vi "Experiments UI.vi"() -> ()   [LabVIEW 2009, in "UI.lvlib"]
uses:
  UI.lvlib
  database/Experiment.ctl
  database/Block.ctl
  Close Notification.vi
  database/Data Store.lvclass
  database/Database.lvlib
  time/Time.lvlib
panel:
  out "Current Block":T1
  in  "Edit users":bool
  out "Experiment status":string
  in  "Save changes":bool
  out "error out":errorcluster
  in  "Run expt":bool
  in  "Description":string
  in  "Name":string
  in  "Update listbox":bool
  out "Working Set":T2[](array[typedef])
  in  "Reload Working Set":bool
  in  "Update Editor":bool
  in  "Delete":bool
  out "Date/time created":string
  in  "New Experiment":bool
  in  "User":u16(ring)=1 items=["CCLDAS"=1, "LDEX"=2]
  in  "Experiments":i32(listbox)
  # "\"Running\" means all dust events will be marked as belonging to this experiment. \nYou can start and stop the experiment as often as you want."
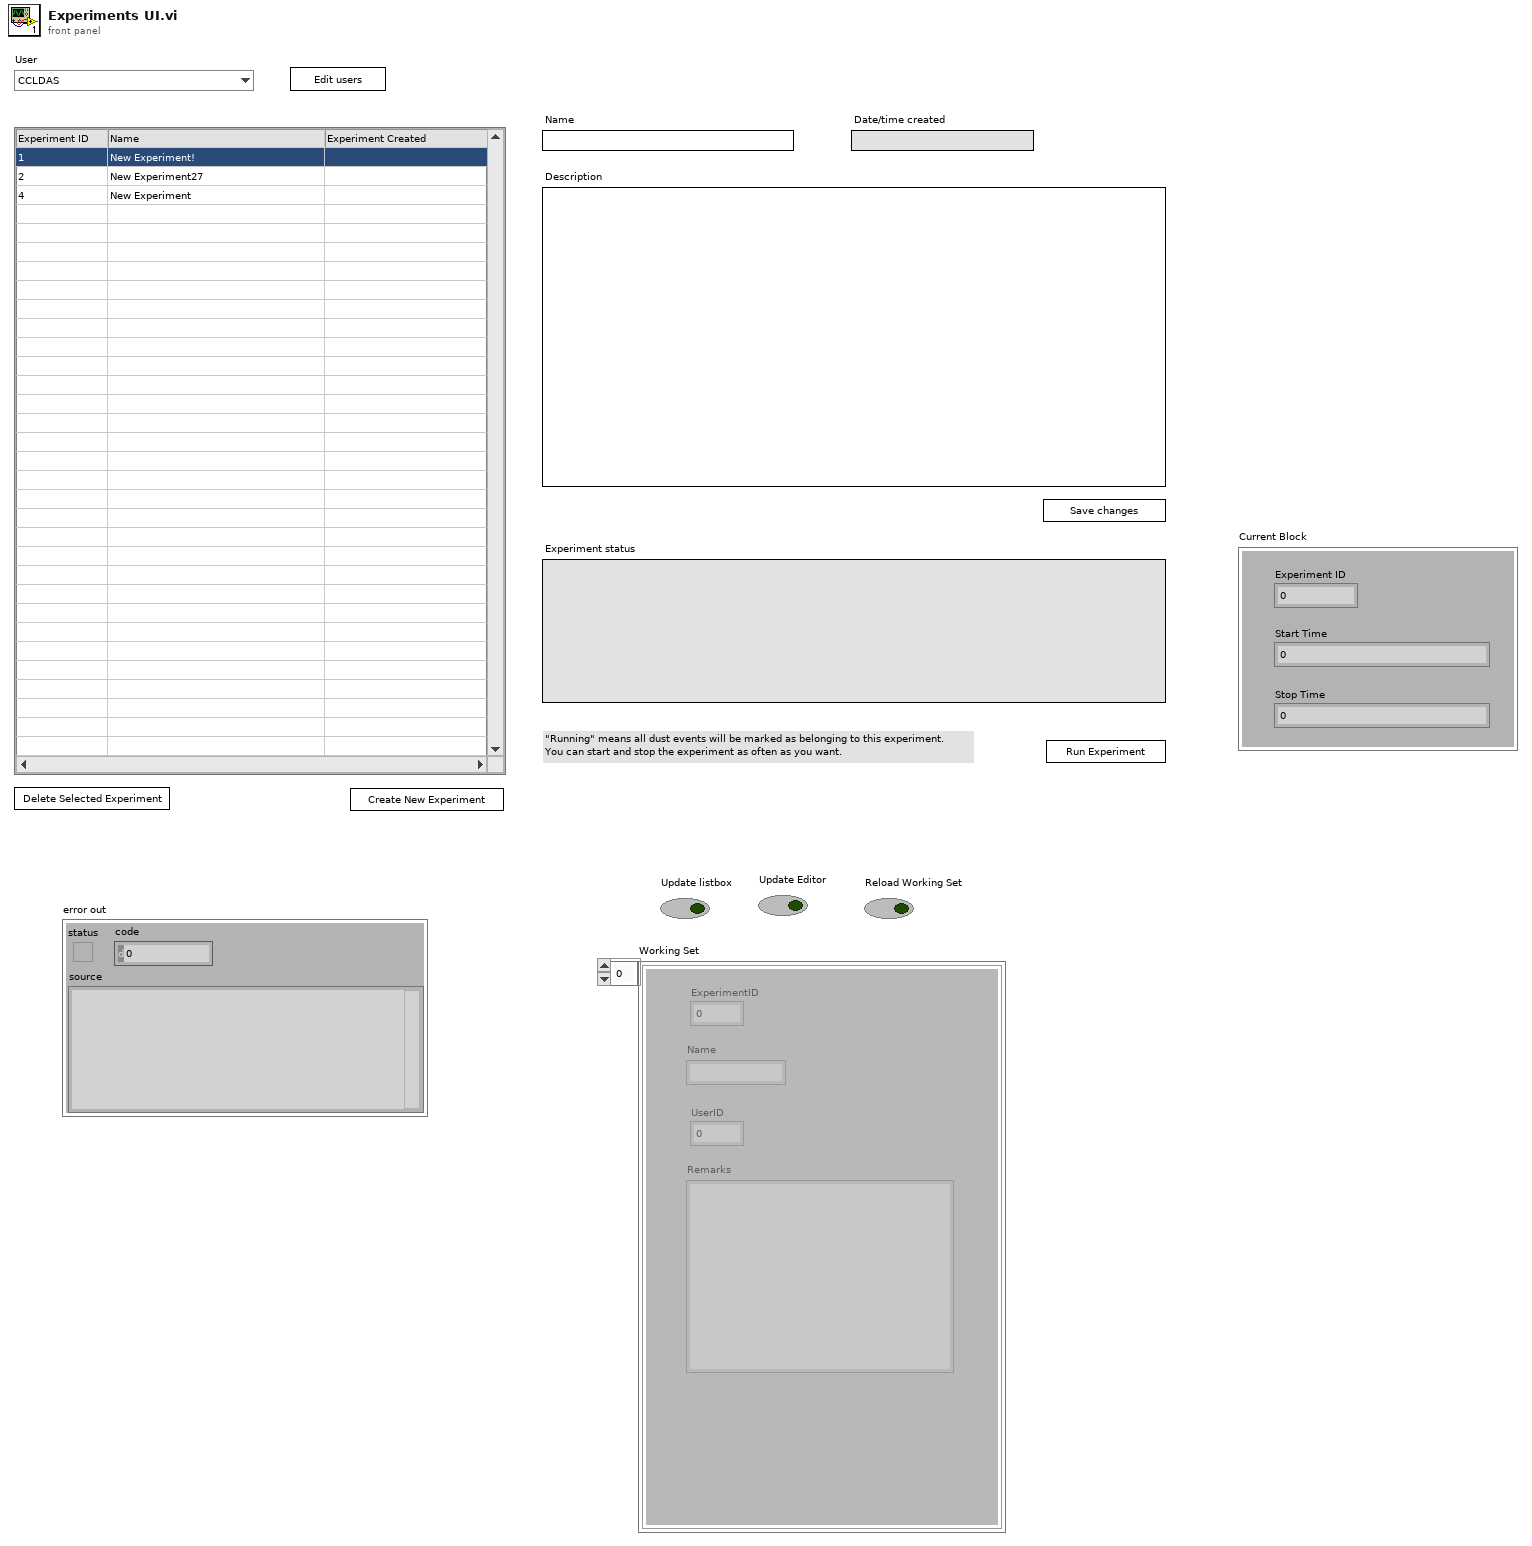
[diagram p1: front panel]
types:
  T1 = typedef "Database.lvlib/Block.ctl" = cluster{"Experiment ID":i32, "Start Time":u64, "Stop Time":u64}
  T2 = typedef "Database.lvlib/Experiment.ctl" = cluster{"ExperimentID":i32, "Name":string, "UserID":i32, "Remarks":string}
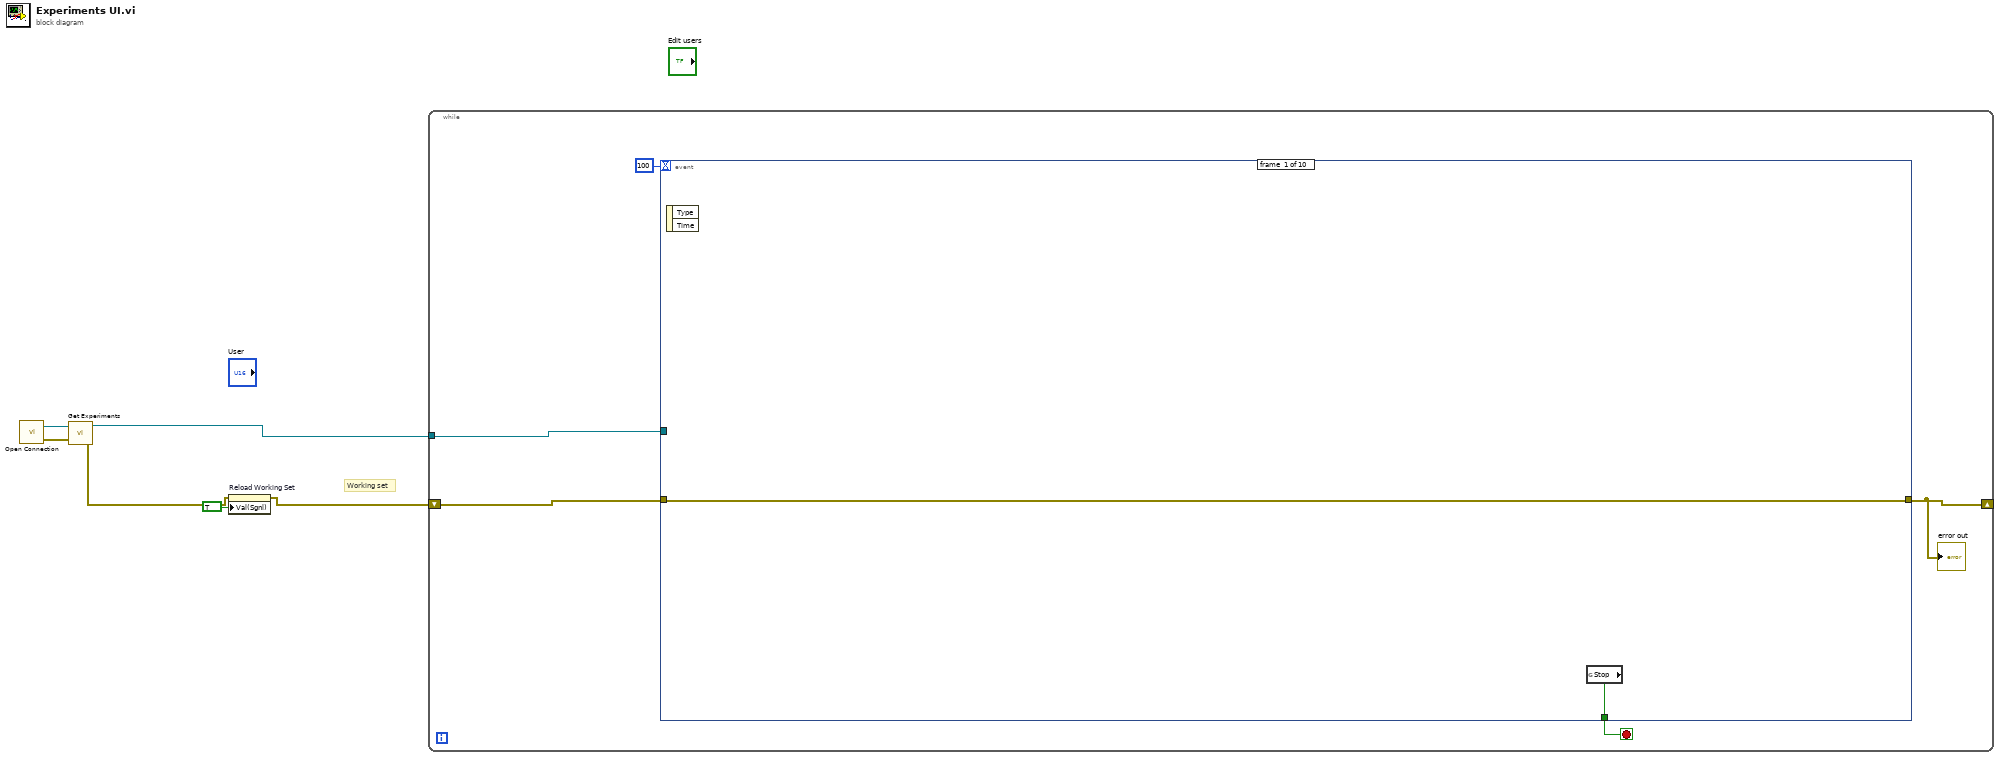
[diagram p0: block diagram]
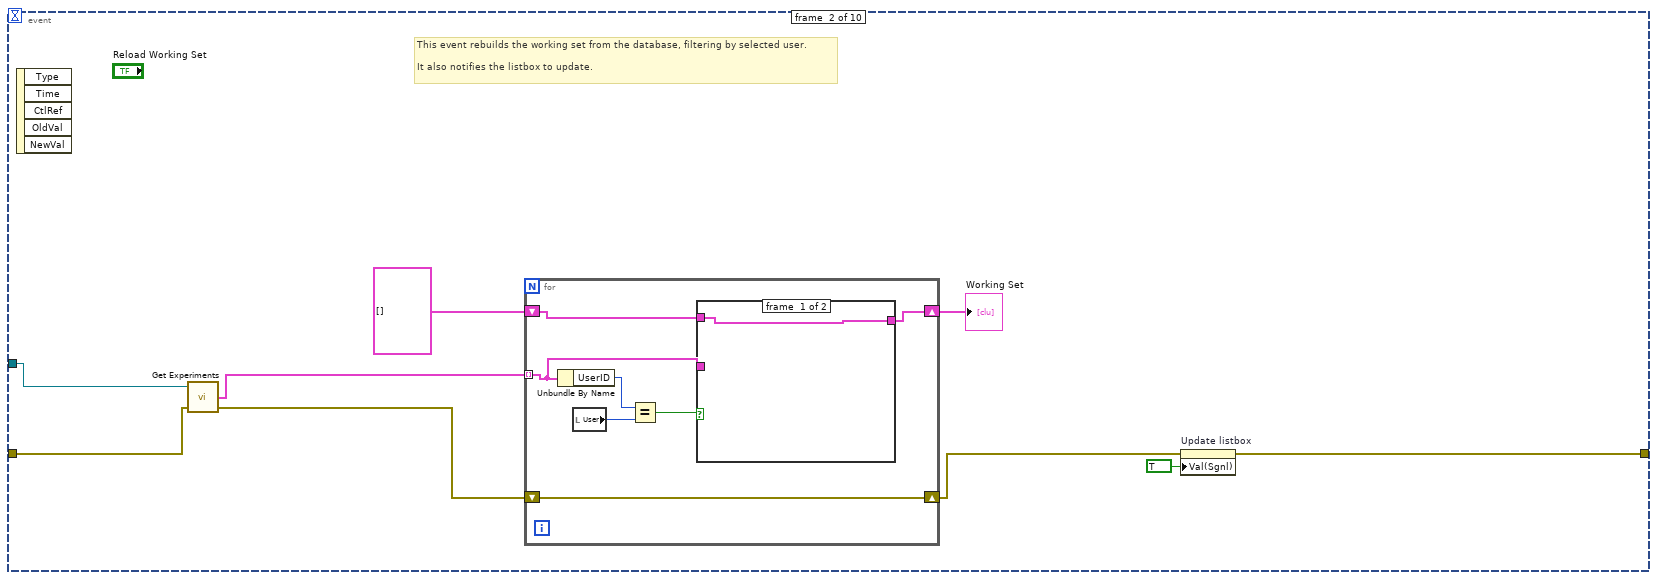
[diagram p2: hidden frame]
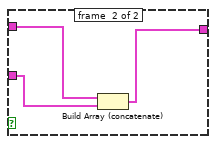
[diagram p3: hidden frame]
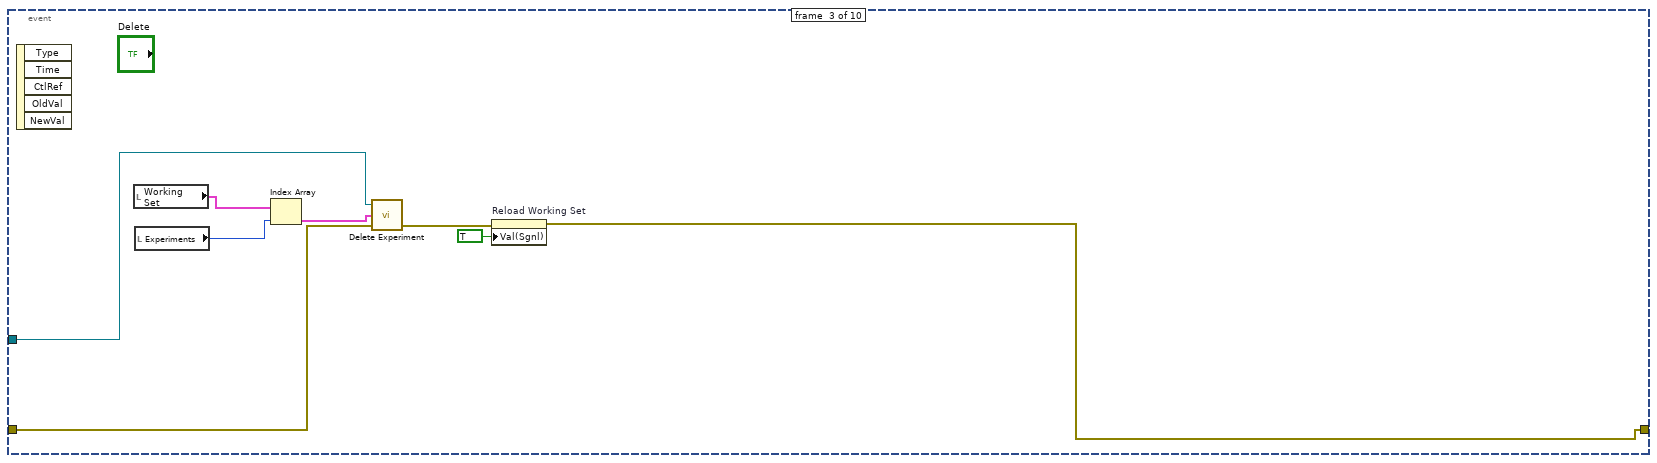
[diagram p4: hidden frame]
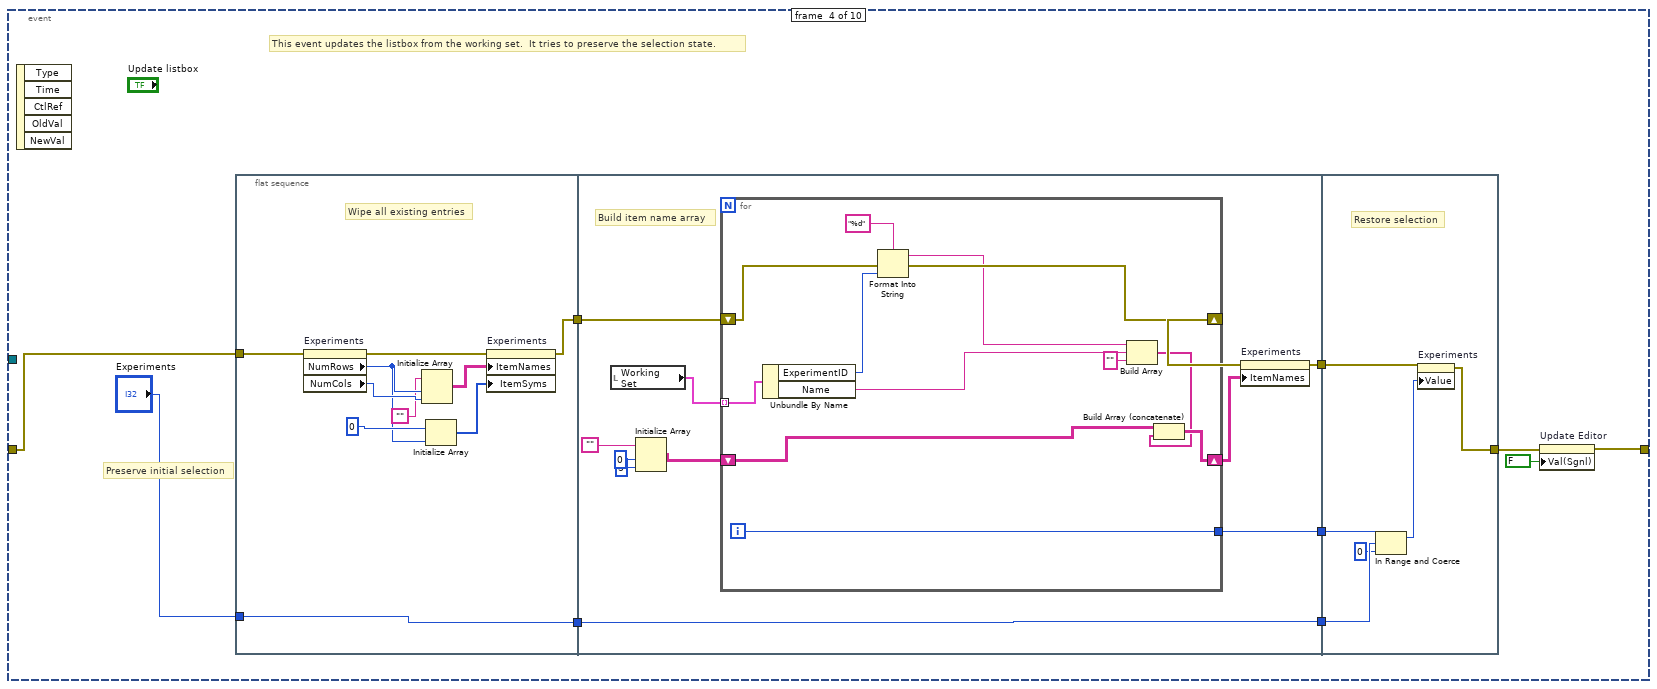
[diagram p5: hidden frame]
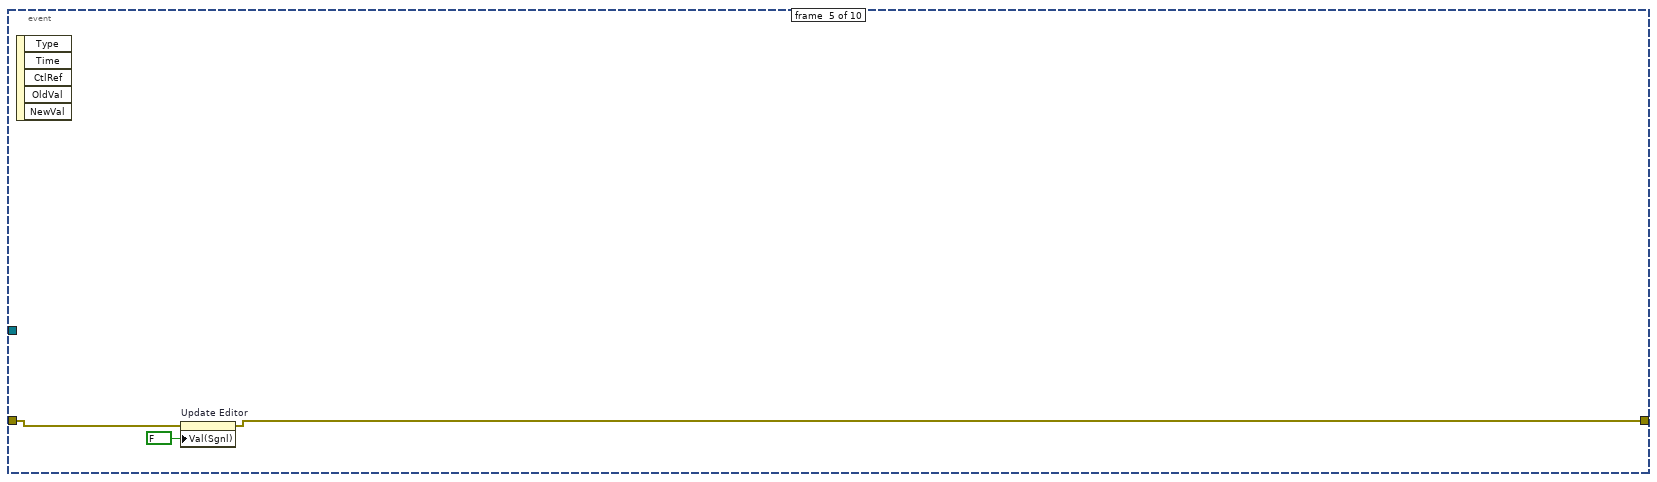
[diagram p6: hidden frame]
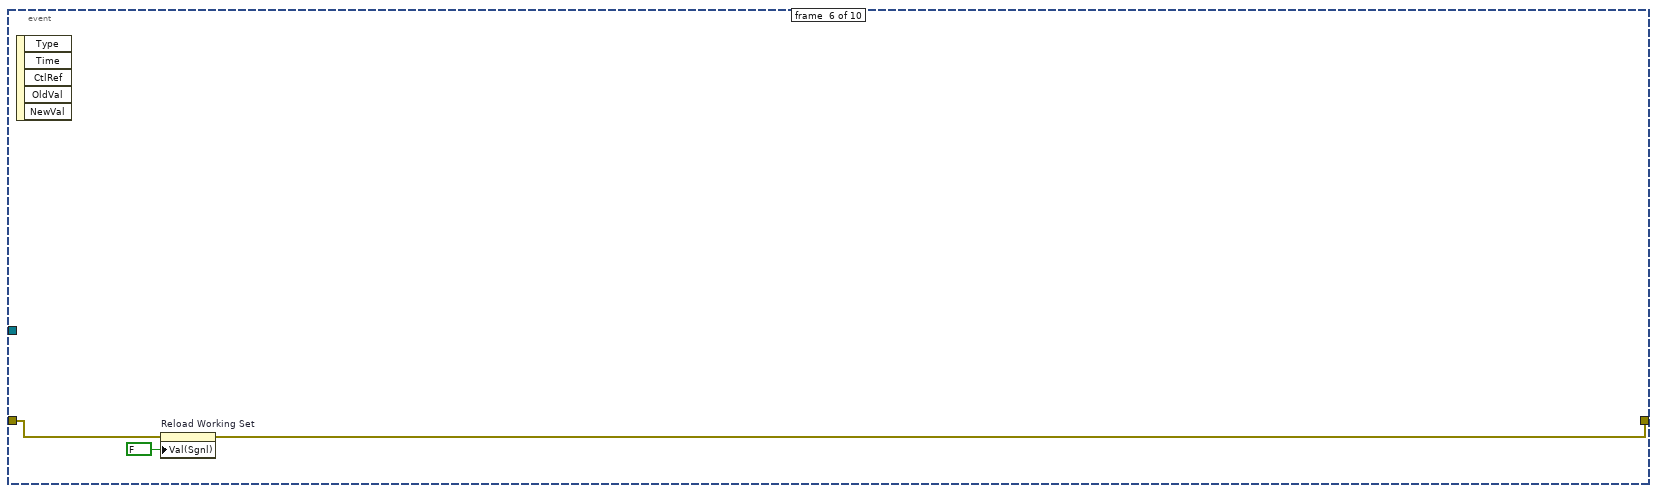
[diagram p7: hidden frame]
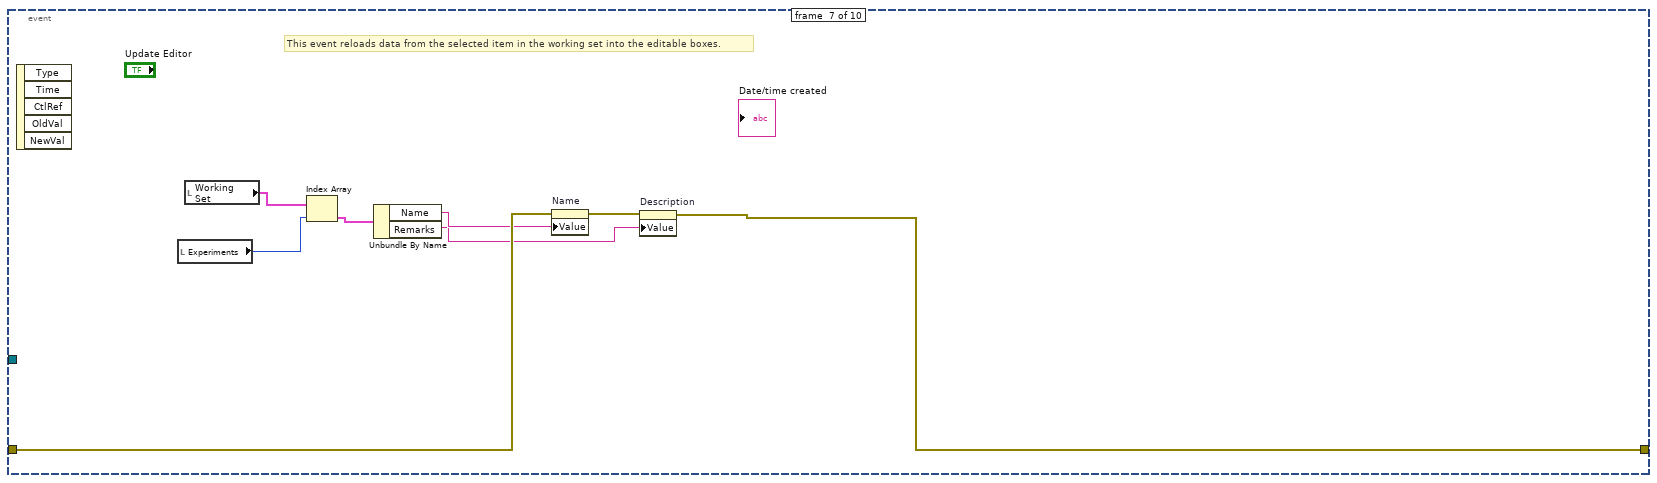
[diagram p8: hidden frame]
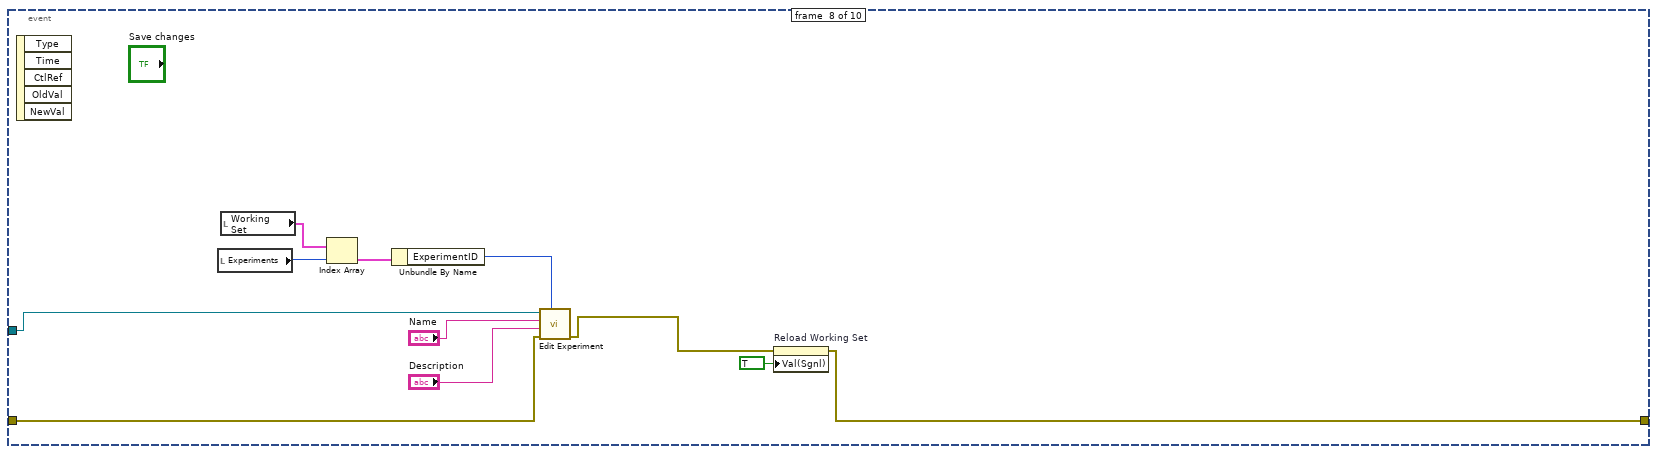
[diagram p9: hidden frame]
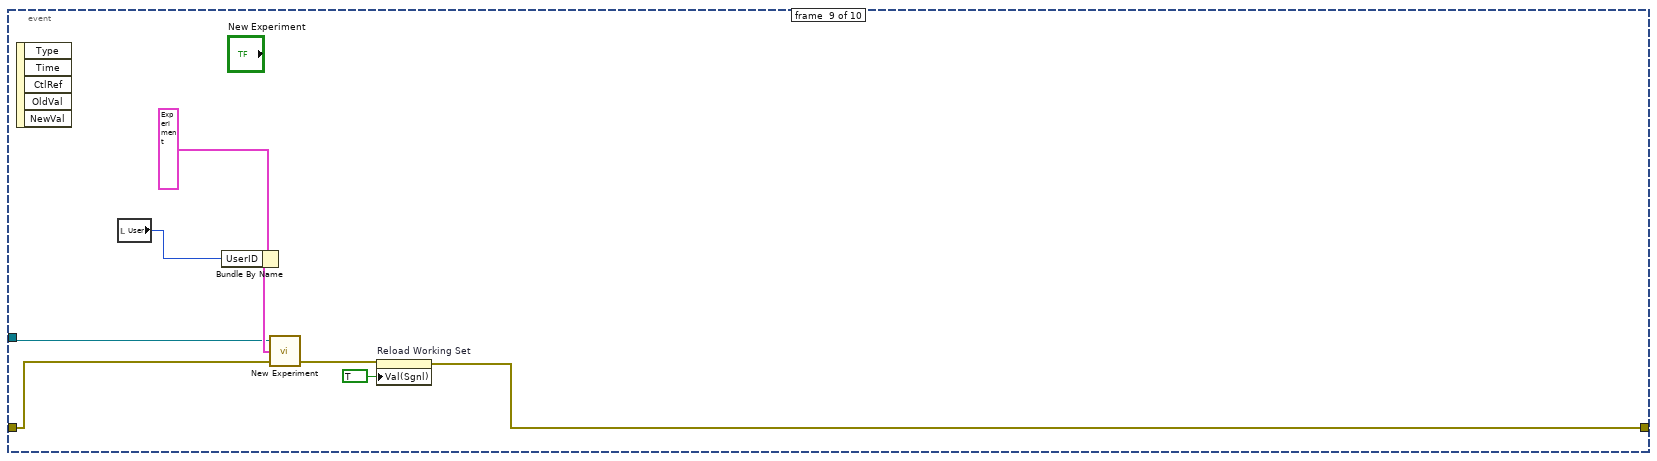
[diagram p10: hidden frame]
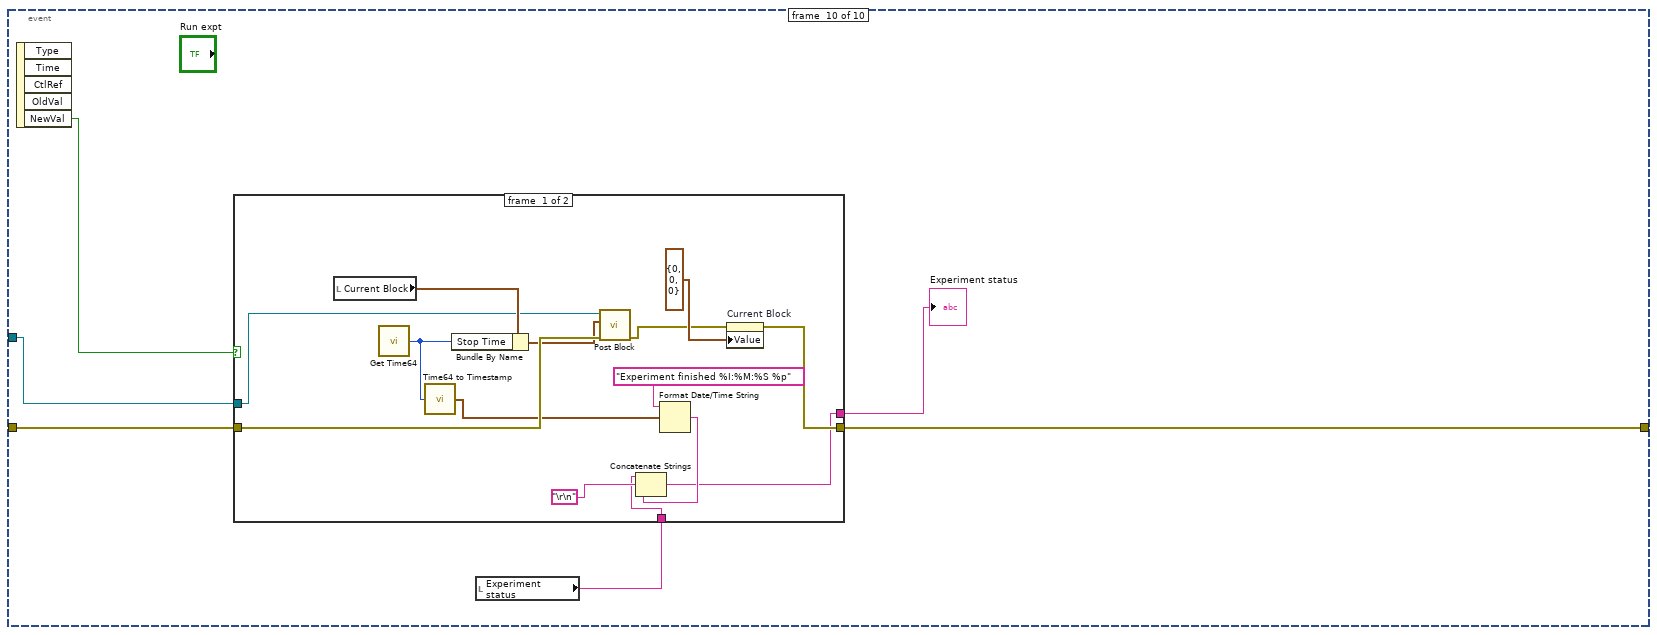
[diagram p11: hidden frame]
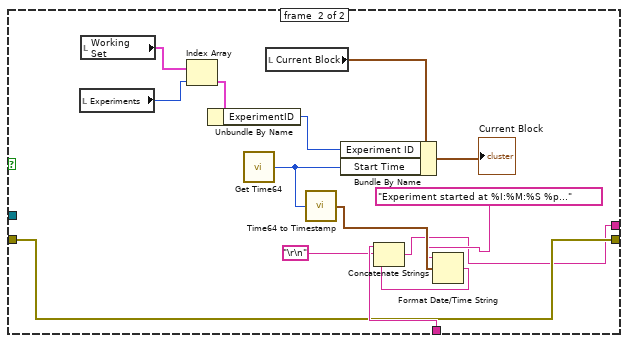
[diagram p12: hidden frame]
diagram:
  # "Working set"
  n1 = call "Open Connection.vi"() -> ("error out"=w6:errorcluster, "Database.lvlib:Data Store.lvclass"=w5:refnum<class "Data Store.lvclass">)  [unwired: 2 in]
  n2 = call "Get Experiments.vi"("error in (no error)"=w6, "Database.lvlib:Data Store.lvclass"=w5) -> ("error out"=w3:errorcluster, "Database.lvlib:Data Store.lvclass 2"=w4:refnum<class "Data Store.lvclass">)  [unwired: 1 in, 1 out]
  n3 = property on="Reload Working Set" class="Bool (strict)"(error in=w3, "Val(Sgnl)"=TRUE ("Value (Signaling)")) -> (error out=w2:errorcluster)  [unwired: 1 in, 1 out]
  n4 = while {
    shift-right: [w7] -> _
    shift-left: w2 -> [w11]
    tunnel: w4 -> [w10]
    stop <- w8 stop-if-true
    n5 = event shown="[9] \"Run expt\": Value Change" {
      selector: _ -> [_ _ _ _ _ _ _ _ _ _]
      dyn-events: _ -> [_ _ _ _ _ _ _ _ _ _]
      timeout: 100 -> [_ _ _ _ _ _ _ _ _ _]
      tunnel: w11 -> [w13 w22 w37 w50 w93 w95 w101 w114 w120 w128]
      tunnel: [w13 w20 w35 w43 w91 w94 w97 w107 w116 w127] -> w7
      tunnel: w10 -> [_ w21 w39 _ _ _ _ w115 w119 w126]
      tunnel: [w12 _ _ _ _ _ _ _ _ _] -> w8
      event #0 {
        n6 = event-data() -> ()  [unwired: 1 in, 2 out]
        n7 = global read "Close Notification.vi" "Stop"() -> (w12:bool)
      }
      event #1 {
        # "This event rebuilds the working set from the database, filtering by selected user.\n\nIt also notifies the listbox to update."
        n8 = event-data() -> ()  [unwired: 1 in, 5 out]
        n9 = call "Get Experiments.vi"("error in (no error)"=w22, "Database.lvlib:Data Store.lvclass"=w21) -> ("error out"=w16:errorcluster, "Array"=w15:T2[])  [unwired: 1 in, 1 out]
        n10 = for {
          shift-right: [w26] -> w17
          shift-left: T2[] [] ("Working Set") -> [w27]
          shift-right: [w23] -> w14
          shift-left: w16 -> [w23]
          tunnel: w15 -> [w24] mode=indexing
          n11 = Unbundle By Name(w24) -> ("UserID"=w29:i32)
          n12 = local read "User"() -> (w28:u16)
          n13 = Equal?(x=w29, y=w28) -> (x = y?=w25:bool)
          n14 = case shown="True" w25 {
            tunnel: w27 -> [w30 w33]
            tunnel: [w30 w31] -> w26
            tunnel: w24 -> [_ w32]
            frame #0 {
            }
            frame #1 {
              n15 = Build Array (concatenate)(w33, w32) -> (w31:T2[])
            }
          }
        }
        "Working Set" <- w17
        n16 = property on="Update listbox" class="Bool (strict)"(error in=w14, "Val(Sgnl)"=TRUE ("Value (Signaling)")) -> (error out=w20:errorcluster)  [unwired: 1 in, 1 out]
      }
      event #2 {
        n17 = event-data() -> ()  [unwired: 1 in, 5 out]
        n18 = local read "Working Set"() -> (w41:T2[])
        n19 = local read "Experiments"() -> (w40:i32)
        n20 = Index Array(array=w41, index=w40) -> (element=w38:T2)
        n21 = call "Delete Experiment.vi"("error in (no error)"=w37, "Experiment to Delete"=w38, "Database.lvlib:Data Store.lvclass"=w39) -> ("error out"=w36:errorcluster)  [unwired: 1 in, 1 out]
        n22 = property on="Reload Working Set" class="Bool (strict)"(error in=w36, "Val(Sgnl)"=TRUE ("Value (Signaling)")) -> (error out=w35:errorcluster)  [unwired: 1 in, 1 out]
      }
      event #3 {
        # "Preserve initial selection"
        # "This event updates the listbox from the working set.  It tries to preserve the selection state."
        n23 = event-data() -> ()  [unwired: 1 in, 5 out]
        n24 = flat-sequence {
          tunnel: "Experiments" -> [w53]
          tunnel: w50 -> [w54]
          tunnel: [w53] -> w49
          tunnel: [w52] -> w48
          tunnel: w49 -> [w72]
          tunnel: w48 -> [w68]
          tunnel: [w72] -> w47
          tunnel: [w64] -> w46
          tunnel: [w63] -> w45
          tunnel: w47 -> [w88]
          tunnel: w46 -> [w90]
          tunnel: w45 -> [w89]
          tunnel: [w85] -> w44
          frame #0 {
            # "Wipe all existing entries"
            n25 = property on="Experiments" class="MCListbox (strict)"(error in=w54) -> (error out=w56:errorcluster, "NumRows"=w57:u32, "NumCols"=w61:u32)  [unwired: 1 in, 1 out]
            n26 = Initialize Array("", w57, w61) -> (w60:string[][])
            n27 = Initialize Array(0, w57) -> (w59:i32[])
            n28 = property on="Experiments" class="MCListbox (strict)"(error in=w56, "ItemNames"=w60, "ItemSyms"=w59) -> (error out=w52:errorcluster)  [unwired: 1 in, 1 out]
          }
          frame #1 {
            # "Build item name array"
            n29 = local read "Working Set"() -> (w67:T2[])
            n30 = Initialize Array("", 0 ("dimension size"), 3 ("dimension size")) -> (w69:string[][])
            n31 = for {
              tunnel: w67 -> [w84] mode=indexing
              shift-right: [w80] -> w65
              shift-left: w68 -> [w82]
              shift-right: [w78] -> w66
              shift-left: w69 -> [w79]
              tunnel: [w74] -> w63
              i -> [w74]
              n32 = Unbundle By Name(w84) -> ("ExperimentID"=w83:i32, "Name"=w81:string)
              n33 = Format Into String(format string="%d", error in=w82, w83) -> (resulting string=w76:string, error out=w80:errorcluster)  [unwired: 1 in]
              n34 = Build Array(w76, w81, "" ("element")) -> (w75:string[])
              n35 = Build Array (concatenate)(w79, w75) -> (w78:string[][])
            }
            n36 = property on="Experiments" class="MCListbox (strict)"(error in=w65, "ItemNames"=w66) -> (error out=w64:errorcluster)  [unwired: 1 in, 1 out]
          }
          frame #2 {
            # "Restore selection"
            n37 = In Range and Coerce(upper limit=w89, x=w88, lower limit=0) -> (coerced(x)=w86:i32)  [unwired: 1 out]
            n38 = property on="Experiments" class="MCListbox (strict)"(error in=w90, "Value"=w86) -> (error out=w85:errorcluster)  [unwired: 1 in, 1 out]
          }
        }
        n39 = property on="Update Editor" class="Bool (strict)"(error in=w44, "Val(Sgnl)"=FALSE ("Value (Signaling)")) -> (error out=w43:errorcluster)  [unwired: 1 in, 1 out]
      }
      event #4 {
        n40 = event-data() -> ()  [unwired: 1 in, 5 out]
        n41 = property on="Update Editor" class="Bool (strict)"(error in=w93, "Val(Sgnl)"=FALSE ("Value (Signaling)")) -> (error out=w91:errorcluster)  [unwired: 1 in, 1 out]
      }
      event #5 {
        n42 = event-data() -> ()  [unwired: 1 in, 5 out]
        n43 = property on="Reload Working Set" class="Bool (strict)"(error in=w95, "Val(Sgnl)"=FALSE ("Value (Signaling)")) -> (error out=w94:errorcluster)  [unwired: 1 in, 1 out]
      }
      event #6 {
        # "This event reloads data from the selected item in the working set into the editable boxes."
        n44 = event-data() -> ()  [unwired: 1 in, 5 out]
        n45 = local read "Experiments"() -> (w103:i32)
        n46 = local read "Working Set"() -> (w104:T2[])
        n47 = Index Array(array=w104, index=w103) -> (element=w102:T2)
        n48 = Unbundle By Name(w102) -> ("Name"=w99:string, "Remarks"=w98:string)
        n49 = property on="Name" class="Str"(error in=w101, "Value"=w99) -> (error out=w100:errorcluster)  [unwired: 1 in, 1 out]
        n50 = property on="Description" class="Str"(error in=w100, "Value"=w98) -> (error out=w97:errorcluster)  [unwired: 1 in, 1 out]
      }
      event #7 {
        n51 = event-data() -> ()  [unwired: 1 in, 5 out]
        n52 = local read "Experiments"() -> (w112:i32)
        n53 = local read "Working Set"() -> (w113:T2[])
        n54 = Index Array(array=w113, index=w112) -> (element=w111:T2)
        n55 = Unbundle By Name(w111) -> ("ExperimentID"=w110:i32)
        n56 = call "Edit Experiment.vi"("Experiment ID"=w110, "error in (no error)"=w114, "Remarks"="Description", "Name"="Name", "Database.lvlib:Data Store.lvclass"=w115) -> ("error out"=w105:errorcluster)  [unwired: 3 in, 1 out]
        n57 = property on="Reload Working Set" class="Bool (strict)"(error in=w105, "Val(Sgnl)"=TRUE ("Value (Signaling)")) -> (error out=w107:errorcluster)  [unwired: 1 in, 1 out]
      }
      event #8 {
        n58 = event-data() -> ()  [unwired: 1 in, 5 out]
        n59 = local read "User"() -> (w122:u16)
        n60 = Bundle By Name(cluster=T2 {"ExperimentID"=0, "Name"="New Experiment", "UserID"=0, "Remarks"=""} ("Cluster"), "UserID"=w122) -> (w121:T2)
        n61 = call "New Experiment.vi"("error in (no error)"=w120, "Experiment in"=w121, "Database.lvlib:Data Store.lvclass"=w119) -> ("error out"=w118:errorcluster)  [unwired: 2 out]
        n62 = property on="Reload Working Set" class="Bool (strict)"(error in=w118, "Val(Sgnl)"=TRUE ("Value (Signaling)")) -> (error out=w116:errorcluster)  [unwired: 1 in, 1 out]
      }
      event #9 {
        n63 = event-data() -> ("NewVal"=w129:bool)  [unwired: 1 in, 4 out]
        n64 = local read "Experiment status"() -> (w125:string)
        n65 = case shown="False" w129 {
          tunnel: [w132 w148] -> w127
          tunnel: w128 -> [w142 w148]
          tunnel: w126 -> [w139 _]
          tunnel: w125 -> [w136 w150]
          tunnel: [w130 w144] -> w124
          frame #0 {
            n66 = local read "Current Block"() -> (w143:T1)
            n67 = call "Get Time64.vi"() -> ("Labview time (ms)"=w137:u64)
            n68 = call "Time64 to Timestamp.vi"("Time64 In"=w137) -> ("Time Stamp"=w133:timestamp)
            n69 = Bundle By Name(cluster=w143, "Stop Time"=w137) -> (w141:T1)
            n70 = call "Post Block.vi"("error in (no error)"=w142, "Cluster"=w141, "Database.lvlib:Data Store.lvclass"=w139) -> ("error out"=w135:errorcluster)  [unwired: 7 in, 1 out]
            n71 = Format Date/Time String(time format string (%c)="Experiment finished %I:%M:%S %p", seconds (now)=w133) -> (date/time string=w131:string)  [unwired: 1 in]
            n72 = Concatenate Strings(w136, "\r\n", w131) -> (w130:string)
            n73 = property on="Current Block" class="Clust (strict)"(error in=w135, "Value"=T1 {"Experiment ID"=0, "Start Time"=0, "Stop Time"=0} ("Current Block")) -> (error out=w132:errorcluster)  [unwired: 1 in, 1 out]
          }
          frame #1 {
            n74 = local read "Experiments"() -> (w156:i32)
            n75 = local read "Working Set"() -> (w157:T2[])
            n76 = Index Array(array=w157, index=w156) -> (element=w155:T2)
            n77 = Unbundle By Name(w155) -> ("ExperimentID"=w153:i32)
            n78 = call "Get Time64.vi"() -> ("Labview time (ms)"=w151:u64)
            n79 = local read "Current Block"() -> (w154:T1)
            n80 = call "Time64 to Timestamp.vi"("Time64 In"=w151) -> ("Time Stamp"=w147:timestamp)
            n81 = Bundle By Name(cluster=w154, "Experiment ID"=w153, "Start Time"=w151) -> (→"Current Block":T1)
            n82 = Format Date/Time String(time format string (%c)="Experiment started at %I:%M:%S %p...", seconds (now)=w147) -> (date/time string=w145:string)  [unwired: 1 in]
            n83 = Concatenate Strings(w150, "\r\n", w145) -> (w144:string)
          }
        }
        "Experiment status" <- w124
      }
    }
    "error out" <- w7
  }
